vi "Calc Neighbours.vi"(11 "Set in":set{cluster{i32, i32}}(c389)) -> (3 "Set out":set{cluster{i32, i32}}(c389))   [LabVIEW 2021]
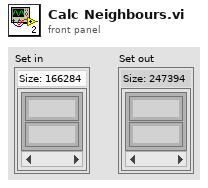
[diagram p1: front panel]
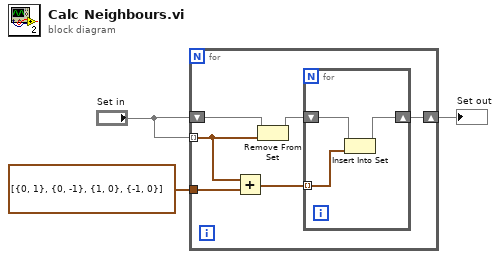
[diagram p0: block diagram]
diagram:
  n1 = for {
    tunnel: cluster{i32, i32}[] [{0, 1}, {0, -1}, {1, 0}, {-1, 0}] -> [w9]
    tunnel: "Set in" -> [w6] mode=indexing
    shift-right: [w8] -> w3
    shift-left: "Set in" -> [w5]
    n2 = Add(x=w6, y=w9) -> (x+y=w7:cluster{i32, i32}[])
    n3 = Remove From Set(10:w6, 11:w5) -> (3:w4:set{cluster{i32, i32}})  [unwired: 1 out]
    n4 = for {
      tunnel: w7 -> [w10] mode=indexing
      shift-right: [w11] -> w8
      shift-left: w4 -> [w12]
      n5 = Insert Into Set(10:w10, 11:w12) -> (3:w11:set{cluster{i32, i32}})  [unwired: 1 out]
    }
  }
  "Set out" <- w3
